vi "Latihan 3 (Tab Control).vi"() -> ()   [LabVIEW 2021]
panel:
  in  "Farenheit":enum32{"Farenheit"}(tab)
  in  "?":dbl(slide) scale=32.0..212.0
  in  "Celcius/Kelvin/Reamur":enum32{" Celcius", "Kelvin", "Reamur"}(tab)
  out "?":dbl(slide) scale=0.0..100.0
  out "?":dbl(slide) scale=273.15..373.15
  out "?":dbl(slide) scale=0.0..80.0
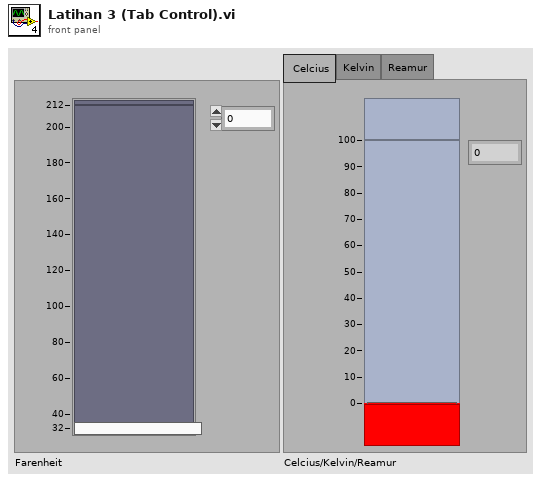
[diagram p1: front panel]
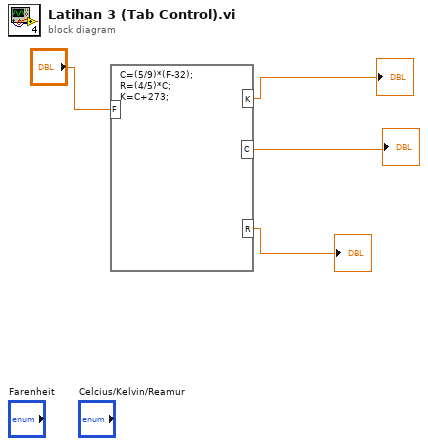
[diagram p0: block diagram]
diagram:
  n1 = formula code="C=(5/9)*(F-32);\nR=(4/5)*C;\nK=C+273;"("F"="?") -> ("C"=→"?":dbl, "R"=→"?":dbl, "K"=→"?":dbl)
